vi "redimensionare imagini.vi"(11 "Cale catre Imagine":path) -> (0 "imagine 28x28":dbl[][](array[numeric]), 1 "Nr Inputs":i32, 2 "Dimensiune imagine":i32[](array[numeric]), 3 "Image 1D Array":dbl[](array[numeric]))   [LabVIEW 2024]
uses:
  <vilib>/vision/NI_Vision_Development_Module.lvlib
panel:
  out "Image":T1(plugin-control)
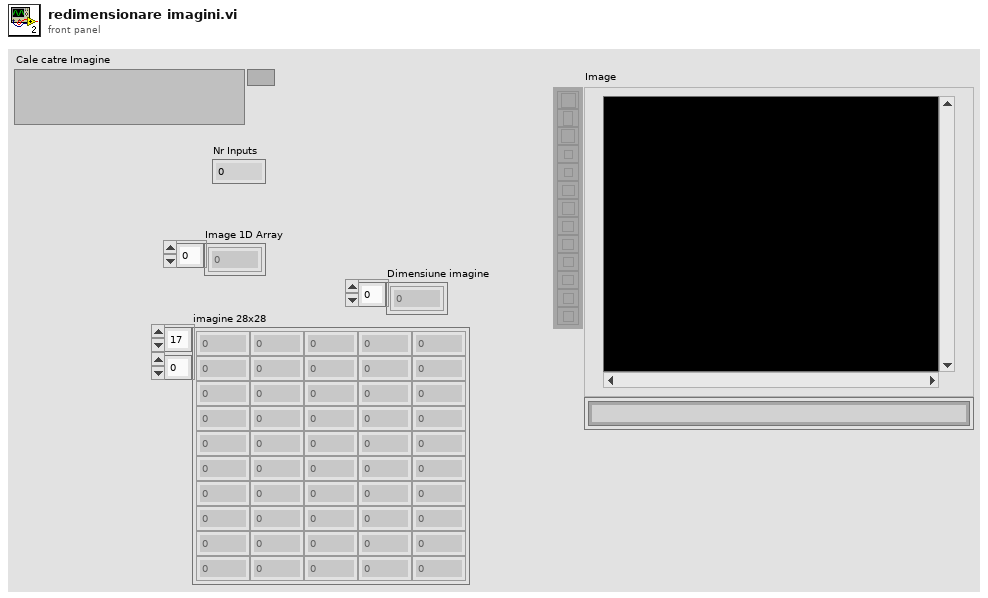
[diagram p1: front panel]
types:
  T1 = typedef "IMAQ Image.ctl" = refnum<image>
  T2 = typedef "Image Type" = u32
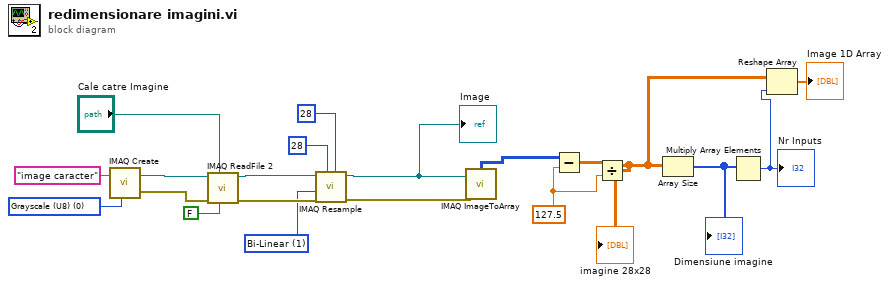
[diagram p0: block diagram]
diagram:
  w5 = 127.5
  w13 = u32 1 items=["Zero Order", "Bi-Linear", "Quadratic", "Cubic Spline"] ("Interpolation Type")
  w17 = T2 0 items=["Grayscale (U8)", "Grayscale (I16)", "Grayscale (SGL)", "Complex (CSG)", "RGB (U32)", "HSL (U32)", "RGB (U64)", "Grayscale (U16)"] ("Image Type")
  n1 = call "IMAQ Create"("Image Name"="image caracter", "Image Type"=w17) -> ("New Image"=w20:T1, "error out"=w16:errorcluster)  [unwired: 3 in]
  n2 = call "IMAQ ReadFile 2"("Use File Path Image Type"=FALSE, "File Path"="Cale catre Imagine", "error in (no error)"=w16, "Image"=w20) -> ("error out"=w15:errorcluster, "Image Out"=w19:T1)  [unwired: 3 in, 3 out]
  n3 = call "IMAQ Resample"("X Resolution"=28, "Y Resolution"=28, "error in (no error)"=w15, "Interpolation Type"=w13, "Image Src"=w19) -> ("error out"=w14:errorcluster, "Image Dst Out"=w8:T1)  [unwired: 5 in]
  "Image" <- w8
  n4 = call "IMAQ ImageToArray"("error in (no error)"=w14, "Image"=w8) -> ("Image Pixels (U8)"=w7:u8[][])  [unwired: 2 in, 4 out]
  n5 = Subtract(x=w7, y=w5) -> (x-y=w6:dbl[][])
  n6 = Divide(x=w6, y=w5) -> (x/y=w3:dbl[][])
  "imagine 28x28" <- w3
  n7 = Array Size(array=w3) -> (size(s)=w4:i32[])
  "Dimensiune imagine" <- w4
  n8 = Multiply Array Elements(1:w4) -> (0:w2:i32)
  "Nr Inputs" <- w2
  n9 = Reshape Array(w3, w2) -> (→"Image 1D Array":dbl[])
